vi "Initialize.vi"(5 "components directory":path, 7 "options":T1, 8 "error in (no error)":errorcluster, 10 "framework configuration":T5, 11 "VeriStand Data Sharing Framework in":refnum<class "VeriStand Data Sharing Framework.lvclass">=refnum) -> (0 "error out":errorcluster, 3 "VeriStand Data Sharing Framework out":refnum<class "VeriStand Data Sharing Framework.lvclass">)   [LabVIEW 2017, in "Data Sharing Framework Engine.lvlib" / "VeriStand Data Sharing Framework.lvclass"]
uses:
  VeriStand Data Sharing Framework.lvclass
  DSF Core.lvlibp/Typedefs/DSF Engine Framework Configuration.ctl
  DSF Core.lvlibp/Typedefs/DSF Engine Plugin Configuration.ctl
  DSF Core.lvlibp/Typedefs/DSF Timing Info.ctl
  DSF Core.lvlibp/Typedefs/DSF Engine Plugin Thread Configuration.ctl
  DSF Core.lvlibp/Typedefs/DSF Settings Info.ctl
  DSF Core.lvlibp/Typedefs/DSF Engine Transfer Group Configuration.ctl
  DSF Core.lvlibp/Typedefs/DSF Direction.ctl
  DSF Core.lvlibp/Typedefs/DSF Engine Transfer Configuration.ctl
  DSF Core.lvlibp/Typedefs/DSF Byte Order.ctl
  DSF Core.lvlibp/Typedefs/DSF Engine Channel Configuration.ctl
  DSF Core.lvlibp/Typedefs/DSF Data Type.ctl
  DSF Core.lvlibp/Classes/Framework/Framework Options.ctl
  DSF Core.lvlibp/Typedefs/DSF FIFO Options.ctl
  DSF Core.lvlibp/Classes/Thread/DSF Thread Options.ctl
  DSF Core.lvlibp/Typedefs/DSF Plugin Options.ctl
  DSF Core.lvlibp/Classes/Framework/Framework.lvclass
  C:/Git/DSF/VeriStand/Data Sharing Custom Device/Source/Engine/DSF Core.lvlibp/Classes/Framework/Framework.lvclass
  DSF Core.lvlibp
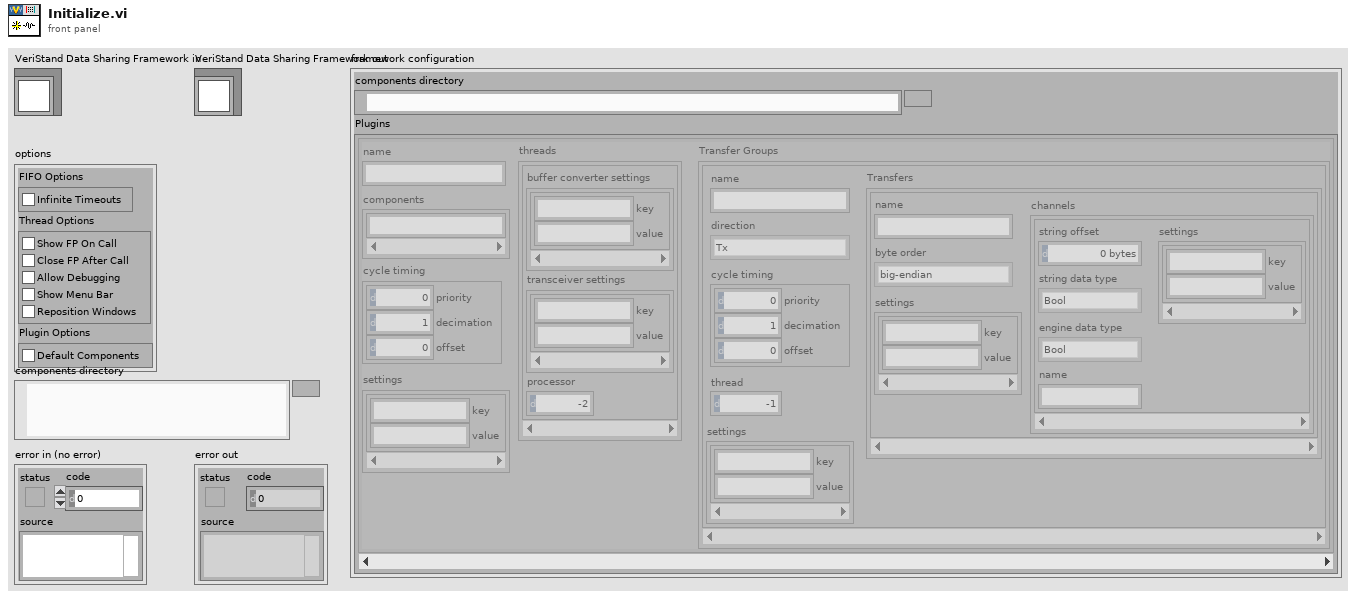
[diagram p1: front panel]
types:
  T1 = typedef "DSF Core.lvlibp/Framework.lvclass/Framework Options.ctl" = cluster{"FIFO Options":T2, "Thread Options":T3, "Plugin Options":T4}
  T2 = typedef "DSF Core.lvlibp/DSF FIFO Options.ctl" = cluster{"Infinite Timeouts":bool}
  T3 = typedef "DSF Core.lvlibp/DSF Thread Options.ctl" = cluster{"Show FP On Call":bool, "Close FP After Call":bool, "Allow Debugging":bool, "Show Menu Bar":bool, "Reposition Windows":bool}
  T4 = typedef "DSF Core.lvlibp/DSF Plugin Options.ctl" = cluster{"Default Components":bool}
  T5 = typedef "DSF Core.lvlibp/DSF Engine Framework Configuration.ctl" = cluster{"components directory":path, "Plugins":T6[]}
  T6 = typedef "DSF Core.lvlibp/DSF Engine Plugin Configuration.ctl" = cluster{"name":string, "components":string[], "cycle timing":T7, "threads":T8[], "Transfer Groups":T10[], "settings":T9}
  T7 = typedef "DSF Core.lvlibp/DSF Timing Info.ctl" = cluster{"priority":u64, "decimation":u64, "offset":u64}
  T8 = typedef "DSF Core.lvlibp/DSF Engine Plugin Thread Configuration.ctl" = cluster{"buffer converter settings":T9, "transceiver settings":T9, "processor":i32}
  T9 = typedef "DSF Core.lvlibp/DSF Settings Info.ctl" = cluster{"key":string, "value":string}[]
  T10 = typedef "DSF Core.lvlibp/DSF Engine Transfer Group Configuration.ctl" = cluster{"name":string, "direction":T11, "cycle timing":T7, "thread":i32, "settings":T9, "Transfers":T12[]}
  T11 = typedef "DSF Core.lvlibp/DSF Direction.ctl" = enum8{"Tx", "Rx"}
  T12 = typedef "DSF Core.lvlibp/DSF Engine Transfer Configuration.ctl" = cluster{"name":string, "byte order":T13, "settings":T9, "channels":T14[]}
  T13 = typedef "DSF Core.lvlibp/DSF Byte Order.ctl" = enum8{"big-endian", "little-endian"}
  T14 = typedef "DSF Core.lvlibp/DSF Engine Channel Configuration.ctl" = cluster{"string offset":u64, "string data type":T15, "engine data type":T15, "name":string, "settings":T9}
  T15 = typedef "DSF Core.lvlibp/DSF Data Type.ctl" = enum8{"Bool", "SGL", "DBL", "I8", "I16", "I32", "I64", "U8", "U16", "U32", "U64"}
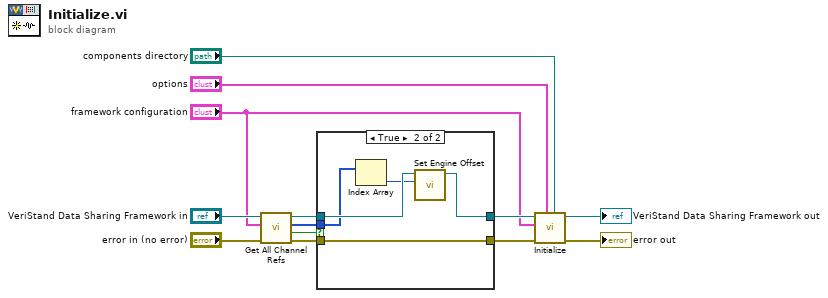
[diagram p0: block diagram]
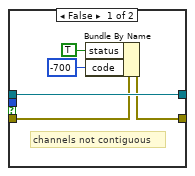
[diagram p2: hidden frame]
diagram:
  n1 = call "Get All Channel Refs.vi"("error in (no error)"="error in (no error)", "framework configuration in"="framework configuration", "VeriStand Data Sharing Framework in"="VeriStand Data Sharing Framework in") -> ("error out"=w10:errorcluster, "contiguous?"=w6:bool, "all channel offsets"=w7:u64[], "VeriStand Data Sharing Framework out"=w8:refnum<class "VeriStand Data Sharing Framework.lvclass">)  [unwired: 5 in]
  n2 = case shown="True" w6 {
    tunnel: [w14 w23] -> w2
    tunnel: [w18 w19] -> w3
    tunnel: w10 -> [w17 w23]
    tunnel: w8 -> [w18 w22]
    tunnel: w7 -> [_ w20]
    frame False {
      # "channels not contiguous"
      n3 = Bundle By Name(cluster=w17, "status"=TRUE, "code"=-700) -> (w14:errorcluster)
    }
    frame True {
      n4 = Index Array(array=w20) -> (element=w21:u64)  [unwired: 1 in]
      n5 = call "Set Engine Offset.vi"("engine offset"=w21, "Framework in"=w22) -> ("Framework out"=w19:refnum<class "VeriStand Data Sharing Framework.lvclass">)  [unwired: 9 in]
    }
  }
  n6 = call-parent "Initialize.vi"("components directory"="components directory", "options"="options", "error in (no error)"=w2, "framework configuration"="framework configuration", "Framework in"=w3) -> ("error out"=→"error out":errorcluster, "Framework out"=→"VeriStand Data Sharing Framework out":refnum<class "VeriStand Data Sharing Framework.lvclass">)  [unwired: 5 in]
